vi "Initialize Attributes.vi"(8 "error in (no error)":errorcluster, 10 "Attribute Data":variant, 11 "CS++DMM in":refnum<class "CS++DMM.lvclass">) -> (0 "error out":errorcluster, 2 "Found?":bool, 3 "CS++DMM out":refnum<class "CS++DMM.lvclass">)   [LabVIEW 2015, in "CS++DMM.lvlib" / "CS++DMM.lvclass"]
doc: "Initialize object attribute.\n\nUnique resources should be allocated elsewhere!"
uses:
  CS++DMM.lvclass
  PV-Enum.ctl
  CSPP_Core/Classes/CS++ProcessVariables/ProcessVariable/PV.lvclass
  CSPP_Core/Classes/CS++ProcessVariables/ProcessVariable/PV.lvclass/PV.ctl
  CSPP_Core/Actors/CS++BaseActor/CS++BaseActor.lvclass/CS++BaseActor.ctl
  CS++DMM.lvclass/CS++DMM.ctl
  CSPP_Core/Classes/CS++ProcessVariables/ProcessVariable/Write PV URL.vi
  CSPP_Core/Classes/CS++ProcessVariables/ProcessVariable/Write Name.vi
  CSPP_Core/Classes/CS++ProcessVariables/ProcessVariable/Write Type Descriptor.vi
  <vilib>/Utility/error.llb/Error Cluster From Error Code.vi
  CSPP_Core/Actors/CS++DeviceActor/CS++DeviceActor.lvclass
  CSPP_Core/Classes/CS++BaseClasses/Factory/CS++Factory.lvclass
  CSPP_Core/Actors/CS++BaseActor/CS++BaseActor.lvclass
  CSPP_Core/Classes/CS++ProcessVariables/CS++ProcessVariables.lvlib
panel:
  in  "PV-Enum":T1=enum."Reading"
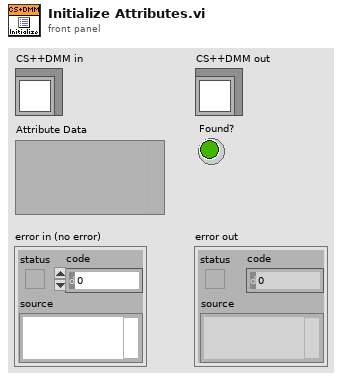
[diagram p1: front panel]
types:
  T1 = typedef "CS++DMM.lvlib/CS++DMM.lvclass/PV-Enum.ctl" = enum16{"AbsoluteResolution", "ACMaxFrequency", "ACMinFrequency", "ActualRange", "Alpha", "ApertureTime", "FixedReferenceJunction", "FrequencyVoltageRange", "PowerLineFrequency", "Range", "Reading", "Resistance", "SampleInterval", "TriggerDelay", "ApertureTimeUnit", "AutoZeroMode", "MeasCompleteDestination", "MeasurementFunction", "ReferenceJunctionType", "SampleCount", "SampleTrigger", "ThermocoupleType", "TranducerType", "TriggerCount", "TriggerSlope", "TriggerSource", "MPReading", "IsOverRange"}
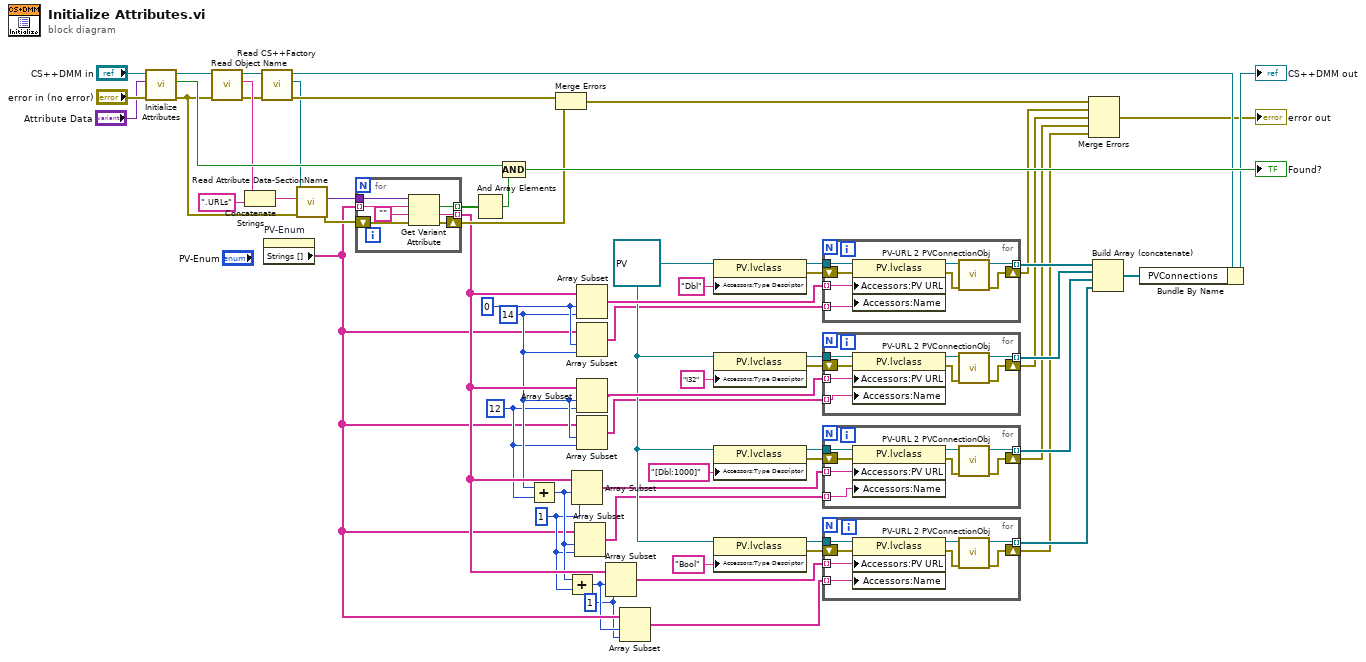
[diagram p0: block diagram]
diagram:
  w2 = 1 ("length")
  w6 = 1 ("length")
  w10 = 12 ("length")
  w11 = 14 ("length")
  w13 = 0 ("index")
  w30 = refnum<class "PV.lvclass"> refnum ("CS++ProcessVariables.lvlib:PV.lvclass")
  n1 = call-parent "Initialize Attributes.vi"("error in (no error)"="error in (no error)", "Attribute Data"="Attribute Data", "CS++DeviceActor in"="CS++DMM in") -> ("error out"=w16:errorcluster, "Found?"=w59:bool, "CS++DeviceActor out"=w56:refnum<class "CS++DMM.lvclass">)  [unwired: 6 in]
  n2 = call "Read Object Name.vi"("error in (no error)"=w16, "CS++BaseActor in"=w56) -> ("error out"=w51:errorcluster, "Object Name"=w55:string, "CS++BaseActor out"=w57:refnum<class "CS++DMM.lvclass">)  [unwired: 7 in]
  n3 = Concatenate Strings(w55, ".URLs" ("string")) -> (w17:string)
  n4 = call "Read CS++Factory.vi"("error in (no error)"=w51, "CS++BaseActor in"=w57) -> ("error out"=w50:errorcluster, "CS++Factory"=w18:refnum<class "CS++Factory.lvclass">, "CS++BaseActor out"=w53:refnum<class "CS++DMM.lvclass">)  [unwired: 7 in]
  n5 = property on="PV-Enum" class="Enum (strict)"() -> ("Strings []"=w4:string[])  [unwired: 2 in, 2 out]
  n6 = call-dynamic "Read Attribute Data-SectionName.vi"("error in (no error)"=w16, "Object Name"=w17, "CS++Factory in"=w18) -> ("error out"=w14:errorcluster, "Attribute Data"=w15:variant)  [unwired: 6 in, 1 out]
  n7 = for {
    tunnel: w15 -> [w68]
    tunnel: w4 -> [w67] mode=indexing
    tunnel: [w64] -> w49 mode=indexing
    tunnel: [w63] -> w31 mode=indexing
    shift-right: [w65] -> w47
    shift-left: w14 -> [w66]
    n8 = Get Variant Attribute(Variant=w68, name=w67, default value (empty Variant)="", error in=w66) -> (found=w64:bool, value=w63:string, error out=w65:errorcluster)  [unwired: 1 out]
  }
  n9 = And Array Elements(Boolean array=w49) -> (logical AND=w48:bool)
  n10 = Compound Arithmetic op=AND(w59, w48) -> (→"Found?":bool)
  n11 = Add(x=w11, y=w10) -> (x+y=w7:i32)
  n12 = Merge Errors(w50, w47) -> (w24:errorcluster)
  n13 = Add(x=w7, y=w6) -> (x+y=w3:i32)
  n14 = Array Subset(array=w31, index=w7, length=w6) -> (w8:string[])
  n15 = Array Subset(array=w4, index=w7, length=w6) -> (w5:string[])
  n16 = Array Subset(array=w31, index=w13, length=w11) -> (w43:string[])
  n17 = Array Subset(array=w4, index=w13, length=w11) -> (w12:string[])
  n18 = Array Subset(array=w31, index=w11, length=w10) -> (w39:string[])
  n19 = Array Subset(array=w4, index=w11, length=w10) -> (w9:string[])
  n20 = Array Subset(array=w31, index=w3, length=w2) -> (w32:string[])
  n21 = Array Subset(array=w4, index=w3, length=w2) -> (w1:string[])
  n22 = property class="PV.lvclass"(reference=w30, "Accessors:Type Descriptor"="Dbl" ("Type Descriptor")) -> (reference out=w45:refnum<class "PV.lvclass">, error out=w46:errorcluster)  [unwired: 1 in]
  n23 = property class="PV.lvclass"(reference=w30, "Accessors:Type Descriptor"="I32" ("Type Descriptor")) -> (reference out=w41:refnum<class "PV.lvclass">, error out=w40:errorcluster)  [unwired: 1 in]
  n24 = property class="PV.lvclass"(reference=w30, "Accessors:Type Descriptor"="[Dbl:1000]" ("Type Descriptor")) -> (reference out=w37:refnum<class "PV.lvclass">, error out=w38:errorcluster)  [unwired: 1 in]
  n25 = property class="PV.lvclass"(reference=w30, "Accessors:Type Descriptor"="Bool" ("Type Descriptor")) -> (reference out=w34:refnum<class "PV.lvclass">, error out=w33:errorcluster)  [unwired: 1 in]
  n26 = for {
    tunnel: w45 -> [w76]
    tunnel: w43 -> [w75] mode=indexing
    tunnel: [w74] -> w29 mode=indexing
    shift-right: [w73] -> w22
    shift-left: w46 -> [w71]
    tunnel: w12 -> [w70] mode=indexing
    n27 = property class="PV.lvclass"(reference=w76, error in=w71, "Accessors:PV URL"=w75, "Accessors:Name"=w70) -> (reference out=w77:refnum<class "PV.lvclass">, error out=w72:errorcluster)
    n28 = call "PV-URL 2 PVConnectionObj.vi"("Error In"=w72, "PV"=w77) -> ("Error Out"=w73:errorcluster, "PVConnection"=w74:refnum<class "PVConnection.lvclass">)  [unwired: 7 in, 1 out]
  }
  n29 = for {
    tunnel: w41 -> [w84]
    tunnel: w39 -> [w83] mode=indexing
    tunnel: [w82] -> w28 mode=indexing
    shift-right: [w81] -> w21
    shift-left: w40 -> [w79]
    tunnel: w9 -> [w78] mode=indexing
    n30 = property class="PV.lvclass"(reference=w84, error in=w79, "Accessors:PV URL"=w83, "Accessors:Name"=w78) -> (reference out=w85:refnum<class "PV.lvclass">, error out=w80:errorcluster)
    n31 = call "PV-URL 2 PVConnectionObj.vi"("Error In"=w80, "PV"=w85) -> ("Error Out"=w81:errorcluster, "PVConnection"=w82:refnum<class "PVConnection.lvclass">)  [unwired: 7 in, 1 out]
  }
  n32 = for {
    tunnel: w37 -> [w92]
    tunnel: w8 -> [w91] mode=indexing
    tunnel: [w90] -> w27 mode=indexing
    shift-right: [w89] -> w20
    shift-left: w38 -> [w87]
    tunnel: w5 -> [w86] mode=indexing
    n33 = property class="PV.lvclass"(reference=w92, error in=w87, "Accessors:PV URL"=w91, "Accessors:Name"=w86) -> (reference out=w93:refnum<class "PV.lvclass">, error out=w88:errorcluster)
    n34 = call "PV-URL 2 PVConnectionObj.vi"("Error In"=w88, "PV"=w93) -> ("Error Out"=w89:errorcluster, "PVConnection"=w90:refnum<class "PVConnection.lvclass">)  [unwired: 7 in, 1 out]
  }
  n35 = for {
    tunnel: w34 -> [w100]
    tunnel: w32 -> [w99] mode=indexing
    tunnel: [w98] -> w26 mode=indexing
    shift-right: [w97] -> w19
    shift-left: w33 -> [w95]
    tunnel: w1 -> [w94] mode=indexing
    n36 = property class="PV.lvclass"(reference=w100, error in=w95, "Accessors:PV URL"=w99, "Accessors:Name"=w94) -> (reference out=w101:refnum<class "PV.lvclass">, error out=w96:errorcluster)
    n37 = call "PV-URL 2 PVConnectionObj.vi"("Error In"=w96, "PV"=w101) -> ("Error Out"=w97:errorcluster, "PVConnection"=w98:refnum<class "PVConnection.lvclass">)  [unwired: 7 in, 1 out]
  }
  n38 = Merge Errors(w24, w22, w21, w20, w19) -> (→"error out":errorcluster)
  n39 = Build Array (concatenate)(w29, w28, w27, w26) -> (w25:refnum<class "PVConnection.lvclass">[])
  n40 = Bundle By Name(cluster=w53, "PVConnections"=w25) -> (→"CS++DMM out":refnum<class "CS++DMM.lvclass">)
